vi "Drive_Set.vi"   [LabVIEW 2019]
uses:
  Drive_Control_States.ctl
  <vilib>/Rock Robotics/WPI/DriverStation/WPI_DriverStationRobotMode2.ctl
  Globals/Drive_Globals.vi
  Robot Global Data.vi
types:
  T1 = typedef "WPI_DriverStationRobotMode2.ctl" = enum16{"Autonomous Disabled", "Autonomous Enabled", "Teleop Disabled", "Teleop Enabled", "Disconnected", "Finish", "Test Disabled", "Test Enabled", "Emergency Stopped"}
  T2 = typedef "Drive_Control_States.ctl" = enum16{"No-Op", "Manual_Control", "Command_DriveDistanceAtAngle", ""}
  T3 = typedef "Drive_Cluster.ctl" = cluster{"Control_State":T2, "Vertical_Throttle":dbl, "Lateral_Throttle":dbl, "Rotational_Throttle":dbl, "Strafe_In_Deadband":bool, "Rotation_In_Deadband":bool, "Orientation_State":T4, "Parameters":dbl[], "Step":i32, "Auto_Notifier":refnum<notifier>}
  T4 = typedef "Drive_Orientation_States.ctl" = enum16{"Robot-Oriented", "Field-Oriented"}
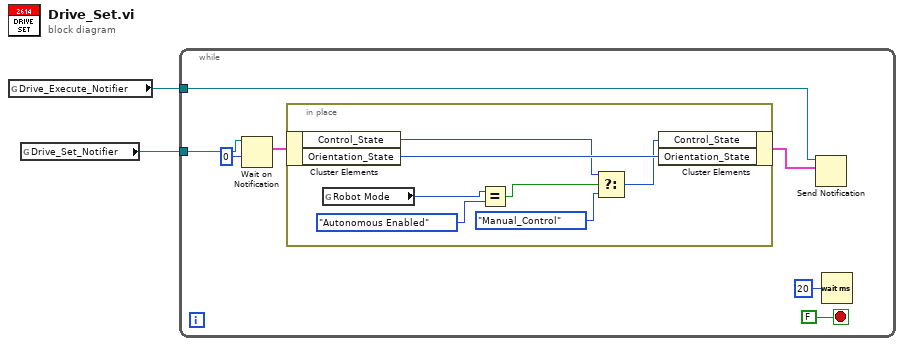
[diagram p0: block diagram]
diagram:
  n1 = global read "Drive_Globals.vi" "Drive_Execute_Notifier"() -> (w2:refnum<notifier>)
  n2 = global read "Drive_Globals.vi" "Drive_Set_Notifier"() -> (w1:refnum<notifier>)
  n3 = while {
    tunnel: w2 -> [w5]
    tunnel: w1 -> [w7]
    stop <- FALSE stop-if-true
    n4 = Wait on Notification(notifier=w7, timeout in ms (-1)=0) -> (notification=w6:T3)  [unwired: 2 in, 3 out]
    n5 = in-place {
      n6 = in-place-cluster #1(w6) -> ("Control_State"=w10:T2, "Orientation_State"=w16:T4)
      n7 = global read "Robot Global Data.vi" "Robot Mode"() -> (w14:T1)
      n8 = Equal?(x=w14, y=WPI_DriverStationRobotMode2."Autonomous Enabled" ("Robot Mode")) -> (x = y?=w13:bool)
      n9 = Select(t=w10, s=w13, f=Drive_Control_States."Manual_Control" ("Control_State")) -> (s? t:f=w12:T2)
      n10 = in-place-cluster #1("Control_State"=w12, "Orientation_State"=w16) -> (w4:T3)
    }
    n11 = Send Notification(notification=w4, notifier=w5) -> ()  [unwired: 1 in, 2 out]
    n12 = Wait (ms)(milliseconds to wait=u32 20) -> ()  [unwired: 1 out]
  }
